vi "ctx v2 mesh data ready.vi"(11 "the_context":u32) -> (2 "function return":i32, 3 "the_context out":u32)   [LabVIEW 2019, in "apdm.lvlib"]
doc: "APDM_EXPORT int apdm_ctx_v2_mesh_data_ready(apdm_ctx_t the_context);"
uses:
  apdm.lvlib
  Lee Lab/CP FES Walking 2018/Code/Working/LabVIEW/apdm.dll
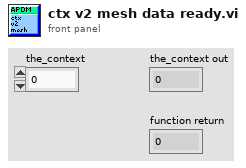
[diagram p1: front panel]
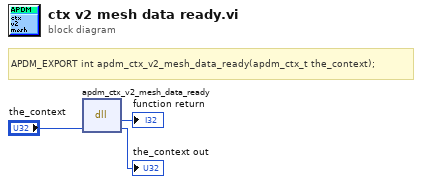
[diagram p0: block diagram]
diagram:
  # "APDM_EXPORT int apdm_ctx_v2_mesh_data_ready(apdm_ctx_t the_context);"
  n1 = dll-call lib="C:/Users/jfalesi/Dropbox/Lee Lab/CP FES Walking 2018/Code/Working/LabVIEW/apdm.*" fn="apdm_ctx_v2_mesh_data_ready"("the_context"="the_context") -> (→"function return":i32, "the_context"=→"the_context out":u32)  [unwired: 3 in, 2 out]
